vi "Write ChannelOn.vi"(8 "error in (no error)":errorcluster, 10 "ChannelOn":bool, 11 "T560Channel in":refnum<class "T560Output.lvclass">) -> (0 "error out":errorcluster, 3 "T560Channel out":refnum<class "T560Output.lvclass">)   [LabVIEW 2020, in "T560Output.lvclass"]
uses:
  T560Output.lvclass
  T560Output.lvclass/T560Output.ctl
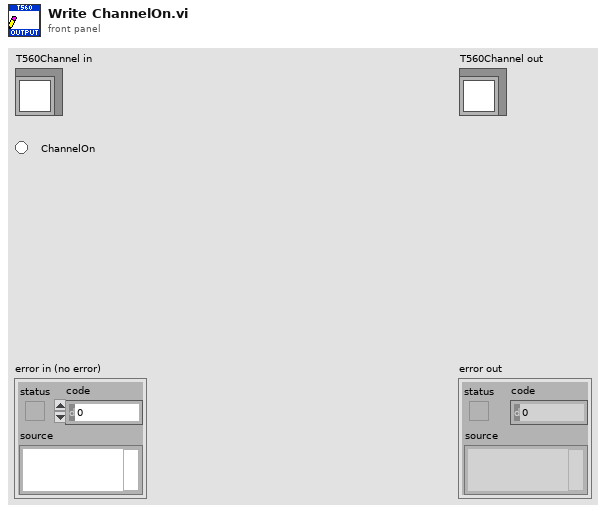
[diagram p1: front panel]
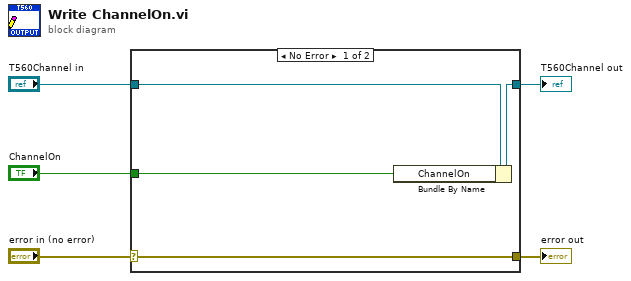
[diagram p0: block diagram]
diagram:
  n1 = case shown="No Error" "error in (no error)" {
    selector: "error in (no error)" -> [w9 w10]
    tunnel: [w9 w10] -> w4
    tunnel: [w7 w11] -> w2
    tunnel: "T560Channel in" -> [w8 w11]
    tunnel: "ChannelOn" -> [w6 _]
    frame No Error {
      n2 = Bundle By Name(cluster=w8, "ChannelOn"=w6) -> (w7:refnum<class "T560Output.lvclass">)
    }
    frame Error {
    }
  }
  "error out" <- w4
  "T560Channel out" <- w2
